vi "Get_Dust_Type_for_Live_Plot.vi"(0 "Start Time":timestamp, 3 "error in (no error)":errorcluster) -> (7 "Dust Type":string, 10 "error out":errorcluster)   [LabVIEW 2013]
uses:
  <userlib>/_OpenG.lib/array/array.llb/Reverse 2D Array (Variant)__ogtk.vi
  <vilib>/addons/database/Connection.llb/Conn Execute.vi
  <vilib>/addons/database/Recordset.llb/Rec Fetch Recordset Data (R).vi
  <vilib>/addons/database/Recordset.llb/Rec Destroy - Connection.vi
  <userlib>/_OpenG.lib/array/array.llb/Empty 2D Array (Variant)__ogtk.vi
  <vilib>/addons/database/_DB Variant To Data/Database Variant To Data.xnode
  <vilib>/addons/database/NI_Database_API.lvlib
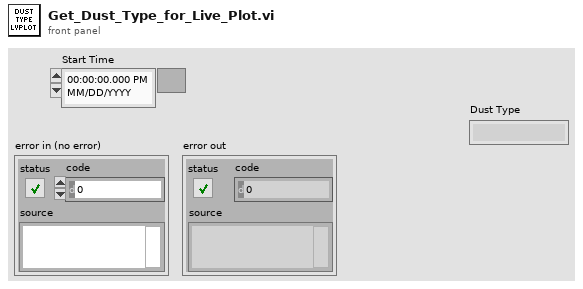
[diagram p1: front panel]
types:
  T1 = typedef "NI_Database_API.lvlib/Conn ObjectReference.ctl" = refnum<k1>
  T2 = typedef "NI_Database_API.lvlib/Rec ObjectReference.ctl" = refnum<k1>
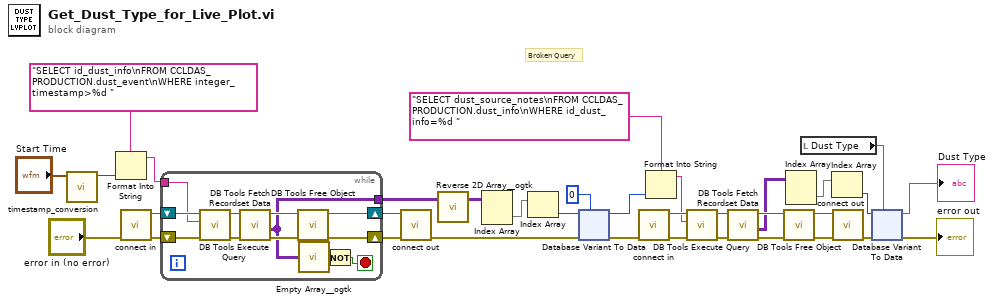
[diagram p0: block diagram]
diagram:
  # "Broken Query"
  n1 = call "timestamp_conversion.vi"("Time Stamp"="Start Time") -> ("Integer Time"=w28:i64)  [unwired: 8 in, 1 out]
  n2 = Format Into String(format string="SELECT id_dust_info\nFROM CCLDAS_PRODUCTION.dust_event\nWHERE integer_timestamp>%d ", w28) -> (resulting string=w27:string)  [unwired: 2 in, 1 out]
  n3 = call "connect in.vi"("error in (no error)"="error in (no error)") -> ("error out"=w33:errorcluster, "Database Connection"=w31:T1)  [unwired: 6 in, 1 out]
  n4 = while {
    shift-right: [w39] -> w32
    shift-left: w33 -> [w41]
    shift-right: [w40] -> w30
    shift-left: w31 -> [w42]
    tunnel: w27 -> [w38]
    tunnel: [w35] -> w21
    stop <- w37 stop-if-true
    n5 = call-poly <vilib>:"DB Tools Execute Query.vi"("error in (no error)"=w41, "SQL query"=w38, "connection reference"=w42) -> ("error out"=w44:errorcluster, "recordset reference"=w45:T2)  [unwired: 5 in]
    n6 = call-poly <vilib>:"DB Tools Fetch Recordset Data.vi"("error in (no error)"=w44, "recordset reference"=w45) -> ("error out"=w43:errorcluster, "recordset data"=w35:variant[][], "recordset reference out"=w46:T2)  [unwired: 3 in]
    n7 = call-poly <vilib>:"DB Tools Free Object.vi"("error in (no error)"=w43, "recordset reference"=w46) -> ("error out"=w39:errorcluster, "connection reference"=w40:T1)  [unwired: 8 in]
    n8 = call-poly <userlib>:"Empty Array__ogtk.vi"("Array"=w35) -> ("Empty Array?"=w36:bool)  [unwired: 8 in]
    n9 = Not(x=w36) -> (.not. x?=w37:bool)
  }
  n10 = call "connect out.vi"("error in (no error)"=w32, "connection reference"=w30) -> ("error out"=w24:errorcluster)  [unwired: 9 in]
  n11 = call-poly <userlib>:"Reverse 2D Array__ogtk.vi"("Array"=w21) -> ("Reversed Array"=w20:variant[][])  [unwired: 2 in]
  n12 = Index Array(array=w20) -> (element=w22:variant[])  [unwired: 2 in]
  n13 = Index Array(array=w22) -> (element=w25:variant)  [unwired: 1 in]
  n14 = xnode "Database Variant To Data"("database variant"=w25, "error in (no error)"=w24, "type"=0) -> ("data"=w19:i32, "error out"=w18:errorcluster)
  n15 = call "connect in.vi"("error in (no error)"=w18) -> ("error out"=w17:errorcluster, "Database Connection"=w12:T1)  [unwired: 6 in, 1 out]
  n16 = Format Into String(format string="SELECT dust_source_notes\nFROM CCLDAS_PRODUCTION.dust_info\nWHERE id_dust_info=%d ", w19) -> (resulting string=w11:string)  [unwired: 2 in, 1 out]
  n17 = call-poly <vilib>:"DB Tools Execute Query.vi"("error in (no error)"=w17, "SQL query"=w11, "connection reference"=w12) -> ("error out"=w16:errorcluster, "recordset reference"=w13:T2)  [unwired: 5 in]
  n18 = call-poly <vilib>:"DB Tools Fetch Recordset Data.vi"("error in (no error)"=w16, "recordset reference"=w13) -> ("error out"=w14:errorcluster, "recordset data"=w1:variant[][], "recordset reference out"=w15:T2)  [unwired: 3 in]
  n19 = call-poly <vilib>:"DB Tools Free Object.vi"("error in (no error)"=w14, "recordset reference"=w15) -> ("error out"=w9:errorcluster, "connection reference"=w8:T1)  [unwired: 8 in]
  n20 = Index Array(array=w1) -> (element=w10:variant[])  [unwired: 2 in]
  n21 = local read "Dust Type"() -> (w4:string)
  n22 = Index Array(array=w10) -> (element=w6:variant)  [unwired: 1 in]
  n23 = call "connect out.vi"("error in (no error)"=w9, "connection reference"=w8) -> ("error out"=w5:errorcluster)  [unwired: 9 in]
  n24 = xnode "Database Variant To Data"("database variant"=w6, "error in (no error)"=w5, "type"=w4) -> ("data"=→"Dust Type":string, "error out"=→"error out":errorcluster)
